vi "Show Animated Busy Icon.vi"(2 "Error In":errorcluster) -> (7 "Error Out":errorcluster)   [LabVIEW 2019]
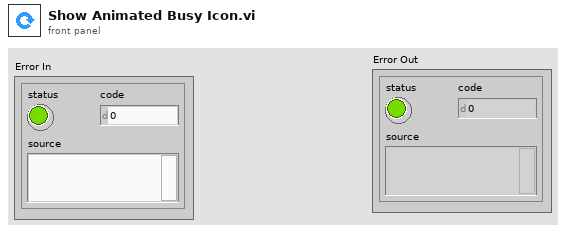
[diagram p1: front panel]
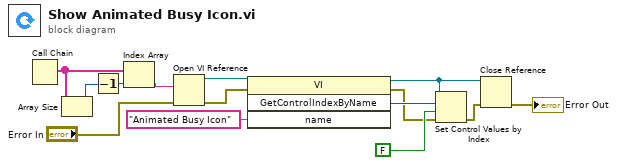
[diagram p0: block diagram]
diagram:
  n1 = Call Chain() -> (call chain=w14:string[])
  n2 = Array Size(array=w14) -> (size(s)=w13:i32)
  n3 = Decrement(x=w13) -> (x-1=w12:i32)
  n4 = Index Array(array=w14, index=w12) -> (element=w11:string)
  n5 = Open VI Reference(vi path=w11, error in (no error)="Error In") -> (vi reference=w5:refnum<vi>, error out=w6:errorcluster)  [unwired: 4 in]
  n6 = invoke class="VI" method="GetControlIndexByName"(reference=w5, error in=w6, "name"="Animated Busy Icon" ("element")) -> (reference out=w4:refnum<vi>, error out=w7:errorcluster, "GetControlIndexByName"=w9:i32)  [unwired: 1 in, 1 out]
  n7 = Set Control Values by Index(0:w4, 1:w9, 2:FALSE ("Visible"), 3:w7) -> (11:w3:errorcluster)
  n8 = Close Reference(reference=w4, error in (no error)=w3) -> (error out=→"Error Out":errorcluster)
